vi "FPGA Main_Scripted_OneNode.vi"() -> ()   [LabVIEW 2014]
uses:
  <vilib>/rvi/Emulation/niFpgaGetClockAttributes.vi
  <vilib>/rvi/Emulation/niFpgaSctlEmulationGetInTimedLoop.vi
  <vilib>/rvi/Emulation/niFpgaEmulationReportErrorSimple.vi
  <vilib>/rvi/Emulation/niFpgaProcessEmulError.vi
  <vilib>/rvi/interface/RandomDataEmulation/niFpgaRandomDataHandleErrors.vi
  <vilib>/rvi/Emulation/niFpgaCriticalErrorInLSC.vi
  <vilib>/rvi/DataTransferAndStorage/Container/XNode/niFpgaContainer.xnode
  <vilib>/rvi/interface/RandomDataEmulation/nirviRandomDataFpgaReadWriteTemplate.vi
  SPIBus0/IO Node Logic Template_SPIBus0.lvlib
panel:
  out "Iteration count":i32
  in  "Debug":bool
  out "FPGA Error":errorcluster
  out "Finished":bool
  in  "stop":bool
  out "Module Underflow":bool
  out "Acq Loop Ticks":u32
  out "DMA FIFO Full":bool
  out "Chan Count":bool
  out "First Read":bool
  in  "Number of Channels":i32=4
  in  "Acquisition Type":enum16{"Finite Samples", "Continuous Samples"}(ring)
  in  "Samps per Chan [Finite]":i32=5120
  in  "Chan Scale Array":sgl[](array[numeric])=[0.0, 0.0, 0.0, 0.0, 0.0, 0.0, 0.0, 0.0, 0.0, 0.0, 0.0, 0.0, 0.0, 0.0, 0.0, 0.0, 0.0, 0.0, 0.0, 0.0, 0.0, 0.0, 0.0, 0.0, 0.0, 0.0, 0.0, 0.0, 0.0, 0.0, 0.0, 0.0, 0.0, 0.0, 0.0, 0.0, 0.0, 0.0, 0.0, 0.0]
  out "oclk mult":u32
  out "oclk div":u32
  out "oclk freq":u32
  in  "data rate (S/s)":u32
  # "Array size fixed at 40\nelements but may be \nexpanded if needed"
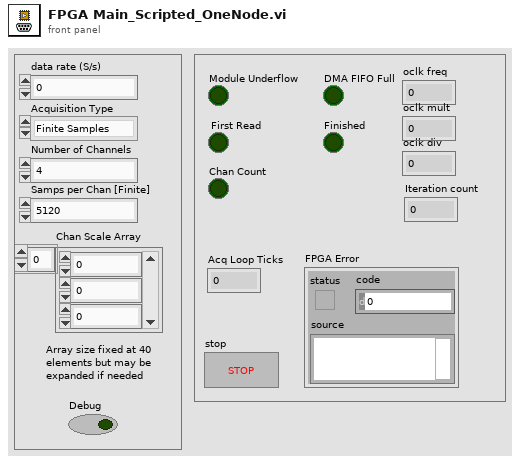
[diagram p1: front panel]
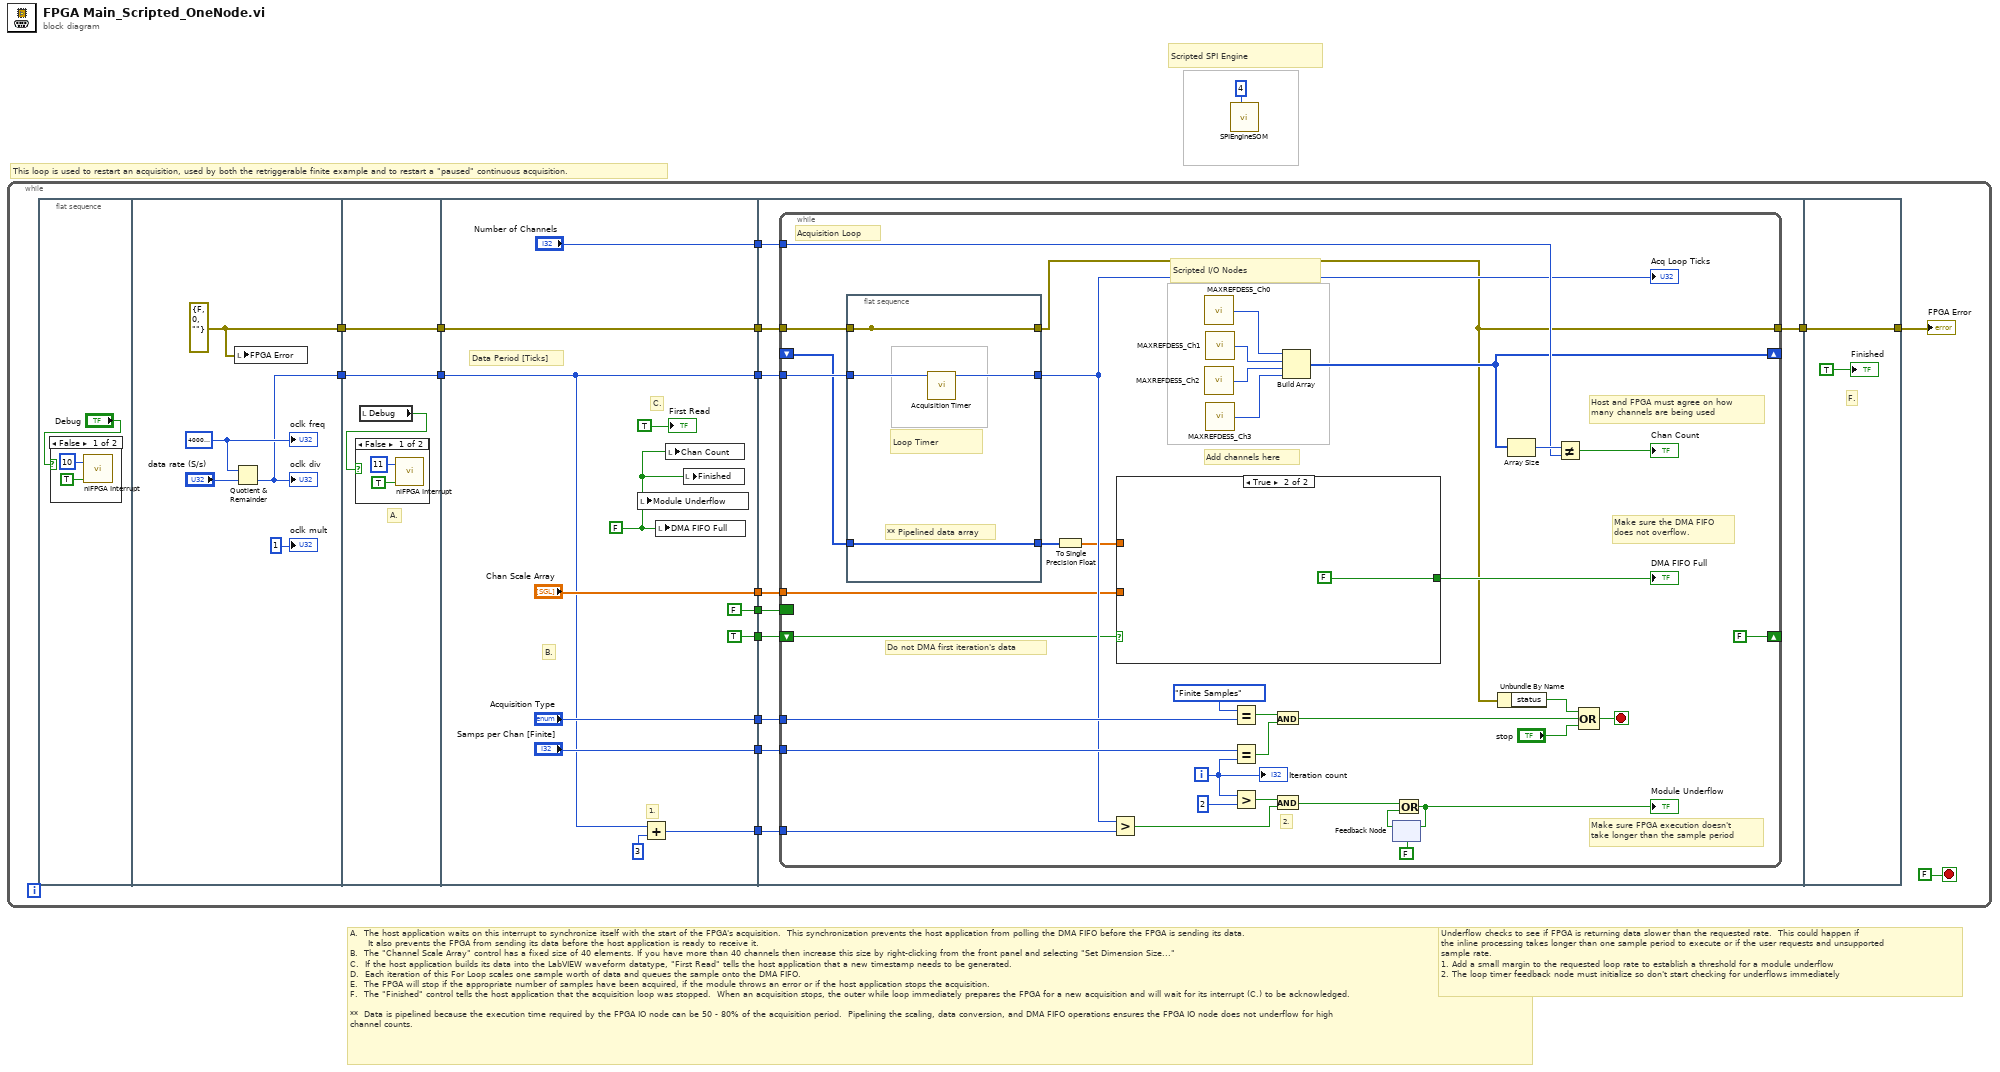
[diagram p0: block diagram]
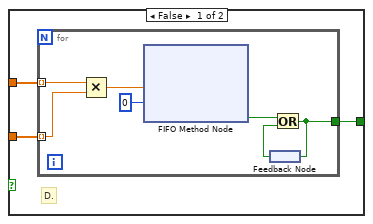
[diagram p4: hidden frame]
diagram:
  # "Scripted SPI Engine"
  # "Underflow checks to see if FPGA is returning data slower than the requested rate.  This could happen if\nthe inline processing takes longer than one sample period to execute or if the user requests and unsupported\nsample rate.\n1. Add a small margin to the requested loop rate to establish a threshold for a module underflow \n2. The loop timer feedback node must initialize so don't start checking for underflows immediately"
  # "A.  The host application waits on this interrupt to synchronize itself with the start of the FPGA's acquisition.  This synchronization prevents the host application from polling the DMA FIFO before the FPGA is sending its data.\n      It also prevents the FPGA from sending its data before the host application is ready to receive it.\nB.  The \"Channel Scale Array\" control has a fixed size of 40 elements. If you have more than 40 channels then increase this size by right-clicking from the front panel and selecting \"Set Dimension Size...\"\nC.  If the host application builds its data into the LabVIEW waveform datatype, \"First Read\" tells the host application that a new timestamp needs to be generated.\nD.  Each iteration of this For Loop scales one sample worth of data and queues the sample onto the DMA FIFO.  \nE.  The FPGA will stop if the appropriate number of samples have been acquired, if the module throws an error or if the host application stops the acquisition.  \nF.  The \"Finished\" control tells the host application that the acquisition loop was stopped.  When an acquisition stops, the outer while loop immediately prepares the FPGA for a new acquisition and will wait for its interrupt (C.) to be acknowledged. \n\n**  Data is pipelined because the execution time required by the FPGA IO node can be 50 - 80% of the acquisition period.  Pipelining the scaling, data conversion, and DMA FIFO operations ensures the FPGA IO node does not underflow for high\nchannel counts."
  # "This loop is used to restart an acquisition, used by both the retriggerable finite example and to restart a \"paused\" continuous acquisition."
  n1 = while {
    stop <- FALSE stop-if-true
    n2 = flat-sequence {
      tunnel: [w22] -> w8
      tunnel: [w21] -> w4
      tunnel: w8 -> [w28]
      tunnel: [w28] -> w7
      tunnel: [w27] -> w5
      tunnel: w4 -> [w27]
      tunnel: ["Number of Channels"] -> w17
      tunnel: ["Chan Scale Array"] -> w16
      tunnel: ["Acquisition Type"] -> w15
      tunnel: ["Samps per Chan [Finite]"] -> w14
      tunnel: [w32] -> w13
      tunnel: [w36] -> w12
      tunnel: [TRUE] -> w11
      tunnel: w7 -> [w33]
      tunnel: [w33] -> w6
      tunnel: w5 -> [w32]
      tunnel: [FALSE] -> w3
      tunnel: w17 -> [w52]
      tunnel: w16 -> [w49]
      tunnel: w15 -> [w48]
      tunnel: w14 -> [w47]
      tunnel: w13 -> [w50]
      tunnel: w12 -> [w46]
      tunnel: w11 -> [w45]
      tunnel: [w44] -> w9
      tunnel: w6 -> [w51]
      tunnel: w3 -> [w43]
      tunnel: [w105] -> w10
      tunnel: w9 -> [w105]
      frame #0 {
        n3 = case shown="False" "Debug" {
          frame False {
            n4 = call <vilib>:"niFPGA Interrupt.vi"("Wait Until Cleared (F)"=TRUE ("Wait Until Cleared"), "IRQ Number (0)"=u8 10 ("IRQ Number")) -> ()  [unwired: 1 in]
          }
          frame True {
          }
        }
      }
      frame #1 {
        w22 = errorcluster {"status"=FALSE, "code"=0, "source"=""} ("FPGA Error")
        w23 = u32 40000000 ("oclk freq")
        n5 = Quotient & Remainder(x=w23, y="data rate (S/s)") -> (floor(x/y)=w21:u32)  [unwired: 1 out]
        "oclk div" <- w21
        n6 = local write "FPGA Error"(w22) -> ()
        "oclk mult" <- u32 1 ("oclk mult")
        "oclk freq" <- w23
      }
      frame #2 {
        # "A."
        n7 = local read "Debug"() -> (w26:bool)
        n8 = case shown="False" w26 {
          frame False {
            n9 = call <vilib>:"niFPGA Interrupt.vi"("Wait Until Cleared (F)"=TRUE ("Wait Until Cleared"), "IRQ Number (0)"=u8 11 ("IRQ Number")) -> ()  [unwired: 1 in]
          }
          frame True {
          }
        }
      }
      frame #3 {
        w41 = FALSE ("Module Underflow")
        # "Data Period [Ticks]"
        # "1."
        # "C."
        # "B."
        n10 = local write "Module Underflow"(w41) -> ()
        n11 = Add(x=w32, y=u32 3) -> (x+y=w36:u32)
        n12 = local write "DMA FIFO Full"(w41) -> ()
        n13 = local write "Chan Count"(w41) -> ()
        n14 = local write "Finished"(w41) -> ()
        "First Read" <- TRUE ("First Read")
      }
      frame #4 {
        n15 = while {
          tunnel: w48 -> [w82]
          tunnel: w47 -> [w81]
          shift-right: [w60] -> _
          shift-left: _ -> [w73]
          tunnel: w52 -> [w83]
          tunnel: w51 -> [w75]
          tunnel: [w56] -> w44
          tunnel: w50 -> [w80]
          tunnel: w46 -> [w76]
          tunnel: w49 -> [w72]
          shift-right: [FALSE] -> _
          shift-left: w45 -> [w71]
          border: w43 -> [_]
          i -> [w69]
          stop <- w87 stop-if-true
          # "Scripted I/O Nodes"
          # "Add channels here"
          # "2."
          # "Do not DMA first iteration's data"
          # "Host and FPGA must agree on how \nmany channels are being used"
          # "Acquisition Loop"
          # "Make sure the DMA FIFO\ndoes not overflow."
          # "Make sure FPGA execution doesn't\ntake longer than the sample period"
          n16 = flat-sequence {
            tunnel: w80 -> [w103]
            tunnel: [w101] -> _
            tunnel: w75 -> [w101]
            tunnel: [w102] -> w74
            tunnel: [w104] -> w59
            tunnel: w73 -> [w104]
            tunnel: [w101] -> w56
            frame #0 {
              # "Loop Timer"
              # "** Pipelined data array"
              n17 = call <vilib>:"Acquisition Timer.vi"("Loop Time (Ticks)"=w103) -> ("Actual Time (Ticks)"=w102:u32)  [unwired: 10 in]
            }
          }
          n18 = To Single Precision Float(number=w59) -> (single precision float=w58:sgl[])
          n19 = Greater?(x=w74, y=w76) -> (0:w79:bool)
          n20 = case shown="True" w71 {
            tunnel: [w92 FALSE] -> w86
            tunnel: w58 -> [w91 _]
            tunnel: w72 -> [w90 _]
            frame False {
              # "D."
              n21 = for {
                tunnel: [w98] -> w92
                tunnel: w91 -> [w97] mode=indexing
                tunnel: w90 -> [w93] mode=indexing
                n22 = Multiply(x=w97, y=w93) -> (x*y=w94:sgl)
                n23 = xnode ("FIFO Method Node")("Element"=w94, "Timeout"=0) -> ("Timed Out?"=w95:bool)  [unwired: 1 in, 1 out]
                n24 = feedback #1() -> (w99:bool)
                n25 = Or(x=w95, y=w99) -> (x .or. y?=w98:bool)
                n26 = feedback-in #1(w98) -> ()
              }
            }
            frame True {
            }
          }
          "DMA FIFO Full" <- w86
          n27 = call "MAXREFDES5_Ch0.vi"() -> ("Received Data"=w57:u64)  [unwired: 15 in]
          n28 = call "MAXREFDES5_Ch2.vi"() -> ("Received Data"=w54:u64)  [unwired: 15 in]
          n29 = call "MAXREFDES5_Ch1.vi"() -> ("Received Data"=w55:u64)  [unwired: 15 in]
          n30 = call "MAXREFDES5_Ch3.vi"() -> ("Received Data"=w53:u64)  [unwired: 15 in]
          n31 = Equal?(x=enum16{"Finite Samples", "Continuous Samples"}."Finite Samples" ("y"), y=w82) -> (x = y?=w63:bool)
          n32 = Equal?(x=w81, y=w69) -> (x = y?=w62:bool)
          n33 = Greater?(x=w69, y=2) -> (0:w78:bool)
          n34 = And(x=w63, y=w62) -> (x .and. y?=w61:bool)
          n35 = And(x=w78, y=w79) -> (x .and. y?=w65:bool)
          n36 = Build Array(w57, w55, w54, w53) -> (w60:u64[])
          n37 = feedback #2(FALSE) -> (w67:bool)
          n38 = Or(x=w65, y=w67) -> (x .or. y?=w64:bool)
          "Module Underflow" <- w64
          n39 = feedback-in #2(w64) -> ()
          n40 = Unbundle By Name(w56) -> ("status"=w68:bool)
          n41 = Array Size(array=w60) -> (size(s)=w85:i32)
          n42 = Not Equal?(x=w85, y=w83) -> (x != y?=→"Chan Count":bool)
          n43 = Compound Arithmetic op=OR(w68, w61, "stop") -> (w87:bool)
          "Acq Loop Ticks" <- w74
          "Iteration count" <- w69
        }
      }
      frame #5 {
        # "F."
        "Finished" <- TRUE ("Finished")
      }
    }
    "FPGA Error" <- w10
  }
  n44 = call "SPIEngineSOM.vi"("NumNodes"=u8 4) -> ()  [unwired: 11 in]
